vi "libssh2_sftp_symlink_ex.vi"(6 "target_len":u32, 7 "link_type":T1, 8 "error in (no error)":errorcluster, 9 "target in":string, 10 "path":string, 11 "sftp":T2) -> (0 "error out":errorcluster, 1 "target out":string)   [LabVIEW 2013, in "libssh2.lvlib"]
doc: "Create a symbolic link or read information about a symbolic link."
uses:
  libssh2.lvlib
  SFTP Refnum.ctl
  libssh2_sftp_symlink_type.ctl
  Not An SFTP Refnum.vi
  <vilib>/Utility/error.llb/Error Cluster From Error Code.vi
  Global Settings.vi
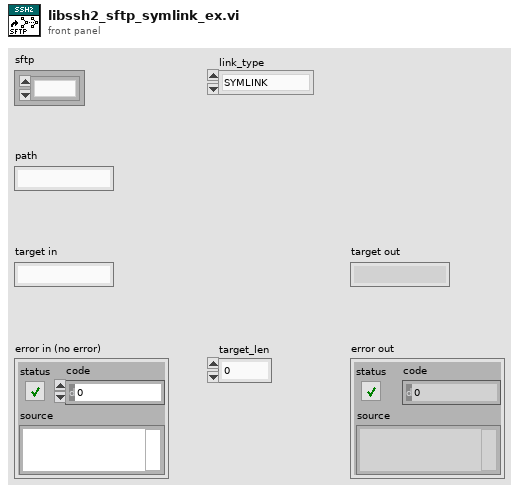
[diagram p1: front panel]
types:
  T1 = typedef "libssh2.lvlib/libssh2_sftp_symlink_type.ctl" = enum16{"SYMLINK", "READLINK", "REALPATH"}
  T2 = typedef "libssh2.lvlib/SFTP Refnum.ctl" = refnum<k1>
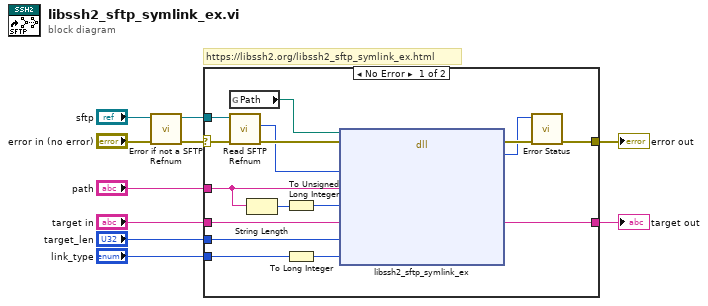
[diagram p0: block diagram]
diagram:
  # "https://libssh2.org/libssh2_sftp_symlink_ex.html"
  n1 = call "Error if not a SFTP Refnum.vi"("error in (no error)"="error in (no error)", "sftp"="sftp") -> ("error out"=w6:errorcluster, "sftp out"=w7:T2)  [unwired: 8 in]
  n2 = case shown="No Error" w6 {
    selector: w6 -> [w25 w27]
    tunnel: w7 -> [w24 _]
    tunnel: [w20 w27] -> w8
    tunnel: "path" -> [w17 _]
    tunnel: "target in" -> [w15 _]
    tunnel: "link_type" -> [w14 _]
    tunnel: [w12 _] -> w2
    tunnel: "target_len" -> [w11 _]
    frame No Error {
      n3 = global read "Global Settings.vi" "Path"() -> (w26:path)
      n4 = call "Read SFTP Refnum.vi"("error in (no error)"=w25, "sftp"=w24) -> ("error out"=w23:errorcluster, "LIBSSH2_SFTP*"=w22:u64)  [unwired: 8 in]
      n5 = String Length(string=w17) -> (length=w18:i32)
      n6 = To Unsigned Long Integer(number=w18) -> (unsigned 32bit integer=w16:u32)
      n7 = To Long Integer(number=w14) -> (32bit integer=w13:i32)
      n8 = dll-call lib="?" fn="libssh2_sftp_symlink_ex"(path in=w26, error in=w23, "sftp"=w22, "path"=w17, "path_len"=w16, "target"=w15, "target_len"=w11, "link_type"=w13) -> (error out=w21:errorcluster, "return value"=w19:i32, "target"=w12:string)  [unwired: 6 in, 1 out]
      n9 = call "Error Status.vi"("error in (no error)"=w21, "return value"=w19) -> ("error out"=w20:errorcluster)  [unwired: 8 in, 1 out]
    }
    frame Error {
    }
  }
  "error out" <- w8
  "target out" <- w2
